vi "Get Reverse Color.vi"(9 "Reverse?":bool, 11 "Color In":u32(colorbox)) -> (3 "Color Out":u32(colorbox))   [LabVIEW 2020, in "2D Plot.lvclass"]
uses:
  <vilib>/Math Plots/2D Math Plots/2D Plot/2D Plot/2D Plot.lvclass
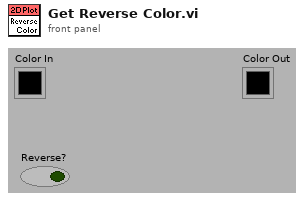
[diagram p1: front panel]
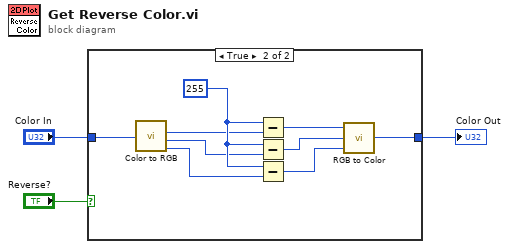
[diagram p0: block diagram]
diagram:
  n1 = case shown="True" "Reverse?" {
    tunnel: "Color In" -> [w4 w13]
    tunnel: [w4 w5] -> w3
    frame False {
    }
    frame True {
      w12 = u8 255 ("x")
      n2 = call <vilib>:"Color to RGB.vi"("Color"=w13) -> ("R"=w9:u8, "G"=w10:u8, "B"=w11:u8)  [unwired: 1 out]
      n3 = Subtract(x=w12, y=w9) -> (x-y=w8:u8)
      n4 = Subtract(x=w12, y=w10) -> (x-y=w7:u8)
      n5 = Subtract(x=w12, y=w11) -> (x-y=w6:u8)
      n6 = call <vilib>:"RGB to Color.vi"("B"=w6, "G"=w7, "R"=w8) -> ("Color"=w5:u32)
    }
  }
  "Color Out" <- w3
